vi "Create Subset Buffers.vi"(6 "inline buffer offset":u64 format="%d bytes", 7 "string buffer offset":u64 format="%d bytes", 8 "error in (no error)":errorcluster, 9 "inline buffer size":u64 format="%d bytes", 10 "string buffer size":u64 format="%d bytes", 11 "Framework in":refnum<class "Framework.lvclass">) -> (0 "error out":errorcluster, 2 "subset Buffers":refnum<class "Buffers.lvclass">, 3 "Framework out":refnum<class "Framework.lvclass">, 4 "inline buffer offset +size":u64 format="%d bytes", 5 "string buffer offset + size":u64 format="%d bytes")   [LabVIEW 2017, in "DSF Core.lvlib" / "Framework.lvclass"]
uses:
  Framework.lvclass
  Buffer/Buffers.lvclass
  Framework.lvclass/Framework.ctl
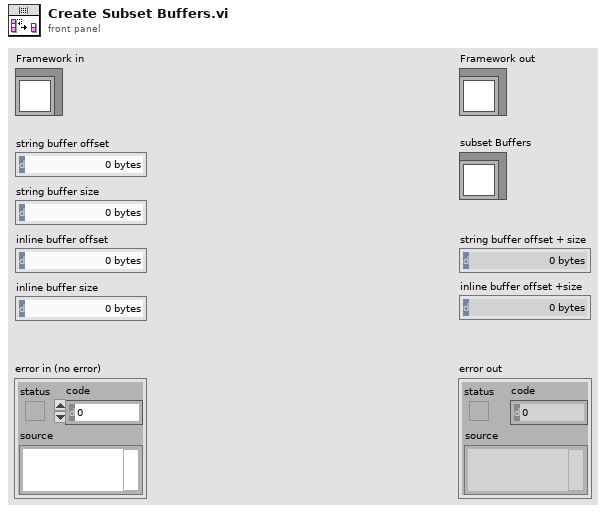
[diagram p1: front panel]
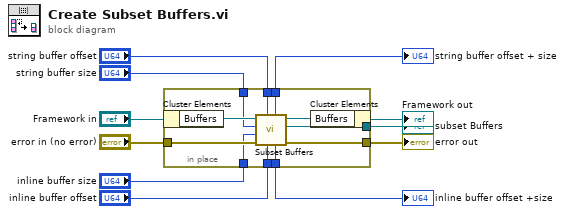
[diagram p0: block diagram]
diagram:
  n1 = in-place {
    in-place-border: "error in (no error)" -> [w22]
    in-place-border: [w21] -> w10
    in-place-border: [w20] -> w9
    in-place-border: "inline buffer size" -> [w17]
    in-place-border: "string buffer size" -> [w16]
    in-place-border: "string buffer offset" -> [w15]
    in-place-border: "inline buffer offset" -> [w14]
    in-place-border: [w13] -> w2
    in-place-border: [w12] -> w1
    n2 = in-place-cluster #1("Framework in") -> ("Buffers"=w19:refnum<class "Buffers.lvclass">)
    n3 = call "Subset Buffers.vi"("inline buffer offset"=w14, "string buffer offset"=w15, "error in (no error)"=w22, "inline buffer size"=w17, "string buffer size"=w16, "Buffers in"=w19) -> ("error out"=w20:errorcluster, "subset Buffers"=w21:refnum<class "Buffers.lvclass">, "Buffers out"=w18:refnum<class "Buffers.lvclass">, "inline buffer offset +size"=w12:u64, "string buffer offset + size"=w13:u64)  [unwired: 1 in]
    n4 = in-place-cluster #1("Buffers"=w18) -> (→"Framework out":refnum<class "Framework.lvclass">)
  }
  "error out" <- w9
  "subset Buffers" <- w10
  "string buffer offset + size" <- w2
  "inline buffer offset +size" <- w1
